vi "String Array 2 Actuator Channels.vi"(1 "Array":string[](array[string])) -> (0 "Actuator Point":T1)   [LabVIEW 2009]
uses:
  Metadata/Actuator Channel Names.ctl
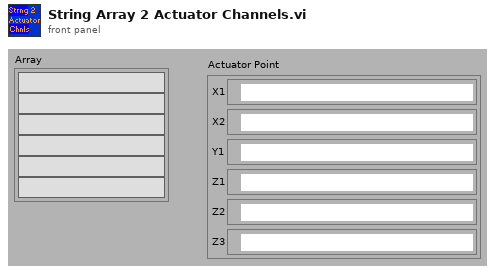
[diagram p1: front panel]
types:
  T1 = typedef "Actuator Channel Names.ctl" = cluster{"X1":refnum<k21>, "X2":refnum<k21>, "Y1":refnum<k21>, "Z1":refnum<k21>, "Z2":refnum<k21>, "Z3":refnum<k21>}
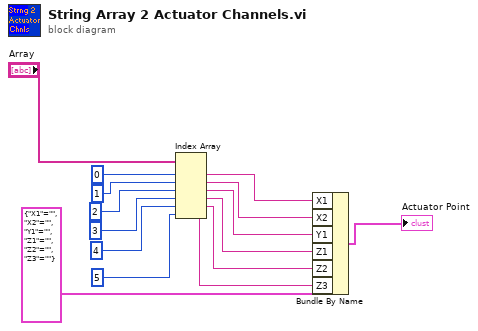
[diagram p0: block diagram]
diagram:
  n1 = Index Array(array="Array", index #1=0 ("index"), index #2=1 ("index"), index #3=2 ("index"), index #4=3 ("index"), index #5=4 ("index"), index #6=5 ("index")) -> (element #1=w8:string, element #2=w9:string, element #3=w10:string, element #4=w11:string, element #5=w12:string, element #6=w13:string)
  n2 = Bundle By Name(cluster=T1 {"X1"="", "X2"="", "Y1"="", "Z1"="", "Z2"="", "Z3"=""} ("Actuator Point"), "X1"=w8, "X2"=w9, "Y1"=w10, "Z1"=w11, "Z2"=w12, "Z3"=w13) -> (→"Actuator Point":T1)
